vi "SeqFrameToJson.vi"(6 "Numeric":i32, 7 "MasterRect":T1, 8 "error in (no error)":errorcluster, 9 "created path":path, 10 "Origin Path":path, 11 "FlatSequenceFrame in":refnum<vi>) -> (0 "error out":errorcluster, 3 "JSON":string)   [LabVIEW 2017]
uses:
  <vilib>/Utility/miscctls.llb/LVRectTypeDef.ctl
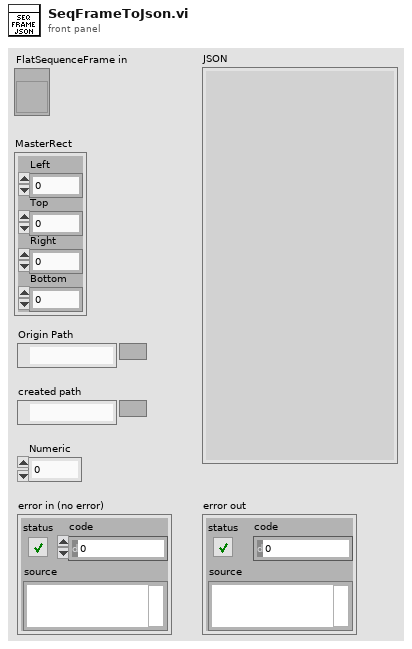
[diagram p1: front panel]
types:
  T1 = typedef "LVRectTypeDef.ctl" = cluster{"Left":i16, "Top":i16, "Right":i16, "Bottom":i16}
  T2 = typedef "LVBoundsTypeDef.ctl" = cluster{"Width":u32, "Height":u32}
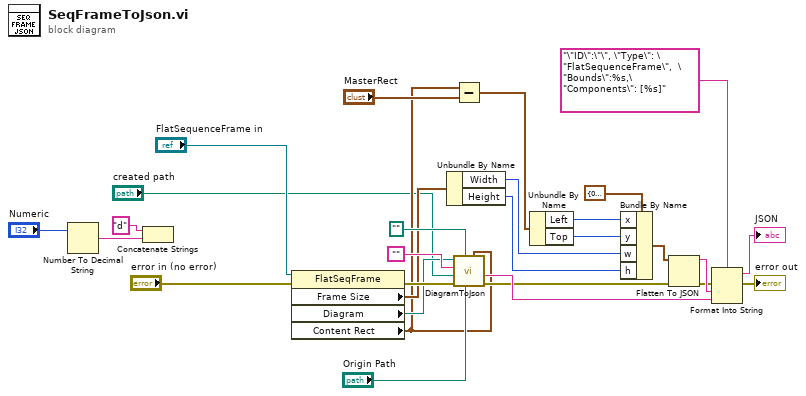
[diagram p0: block diagram]
diagram:
  n1 = Number To Decimal String(number="Numeric") -> (decimal integer string=w16:string)  [unwired: 1 in]
  n2 = Concatenate Strings("d" ("string"), w16) -> ()  [unwired: 1 out]
  n3 = property class="FlatSeqFrame"(reference="FlatSequenceFrame in", error in="error in (no error)") -> (error out=w9:errorcluster, "Frame Size"=w7:T2, "Diagram"=w8:refnum<vi>, "Content Rect"=w2:T1)  [unwired: 1 out]
  n4 = Unbundle By Name(w7) -> ("Width"=w5:u32, "Height"=w4:u32)
  n5 = Subtract(x=w2, y="MasterRect") -> (x-y=w11:T1)
  n6 = call "DiagramToJson.vi"("Owner Bounds"=w2, "Origin Path"="Origin Path", "Image Path"=path "", "error in (no error)"=w9, "Current Path"="created path", "ID"="", "GObj in"=w8) -> ("error out"=w23:errorcluster, "JSON (out)"=w27:string)  [unwired: 2 in, 1 out]
  n7 = Unbundle By Name(w11) -> ("Left"=w12:i16, "Top"=w13:i16)
  n8 = Bundle By Name(cluster=cluster{"x":i32, "y":i32, "w":i32, "h":i32} {"x"=0, "y"=0, "w"=0, "h"=0} ("Rect 2"), "x"=w12, "y"=w13, "w"=w5, "h"=w4) -> (w22:cluster{"x":i32, "y":i32, "w":i32, "h":i32})
  n9 = Flatten To JSON(anything=w22, error in (no error)=w23) -> (JSON string=w26:string, 11:w24:errorcluster)  [unwired: 1 in]
  n10 = Format Into String(format string="\"ID\":\"\", \"Type\": \"FlatSequenceFrame\",  \"Bounds\":%s,\"Components\": [%s]", error in=w24, w26, w27) -> (resulting string=→"JSON":string, error out=→"error out":errorcluster)  [unwired: 1 in]
